vi "GEA2 Serial Dryer Read Write.vi"(0 "Com Chan":u8, 7 "Dryer Status Serial Data In":T1, 11 "error in (no error)":errorcluster) -> (4 "Dryer Status Serial Data":T1, 6 "Read Buffer":string, 8 "Log String":string, 15 "error out":errorcluster)   [LabVIEW 2014]
uses:
  Dryer Wilt/Type Definitions/WILT Dryer Com Port Info.ctl
  Dryer Wilt/Type Definitions/WILT Dryer Status Ctrl.ctl
  Type Definitions/GEA2 Serial Dryer Interface Ctrl.ctl
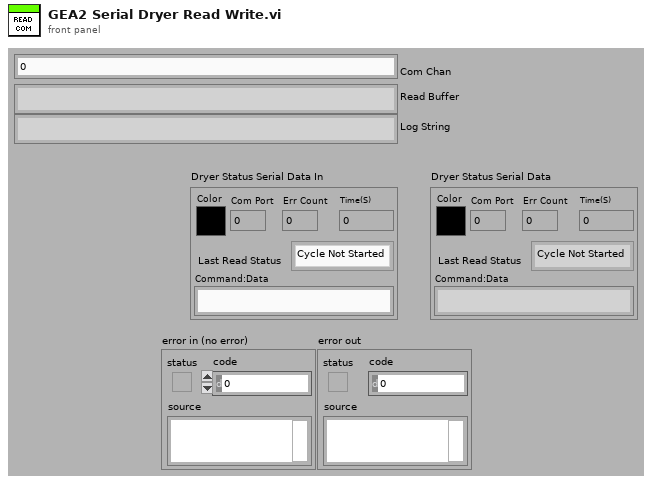
[diagram p1: front panel]
types:
  T1 = typedef "WILT Dryer Com Port Info.ctl" = cluster{"Color":u32, "Last Read Status":T2, "Command:Data":string, "Com Port":u8, "Time(S)":dbl, "Err Count":u32}
  T2 = typedef "WILT Dryer Status Ctrl.ctl" = enum16{"Cycle Not Started", "Cycle Running", "Paused", "Cycle Completed", "Eval Mode Entered", "Err", "Pause (No GEA2)"}
  T3 = typedef "GEA2 Serial Dryer Interface Ctrl.ctl" = enum16{"Init Com Port", "SendCMD", "ReadPort", "Close Port", "Simulate Diag Data", "Send WILT Startup CMDs", "Send Continue CMD", "Read Continuous"}
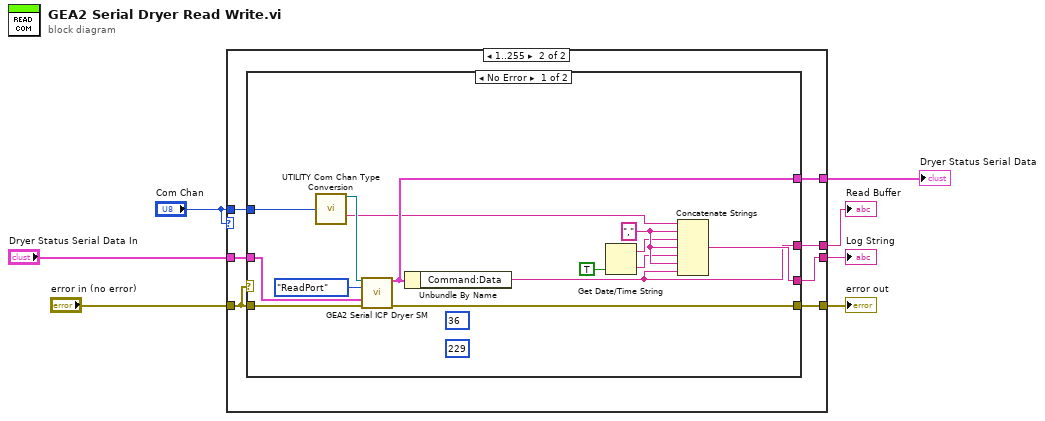
[diagram p0: block diagram]
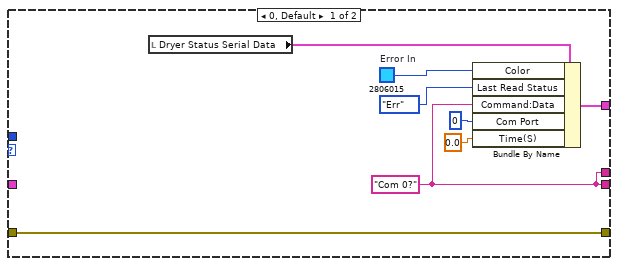
[diagram p2: hidden frame]
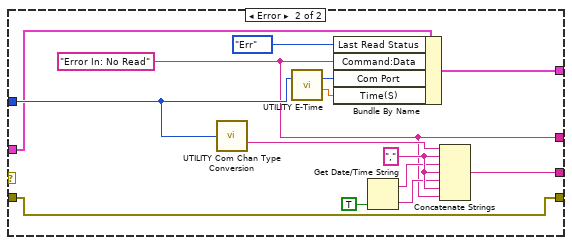
[diagram p3: hidden frame]
diagram:
  n1 = case shown="1..255" "Com Chan" {
    tunnel: "Com Chan" -> [_ w22]
    tunnel: [w15 w21] -> w7
    tunnel: "error in (no error)" -> [w15 w20]
    tunnel: [w11 w19] -> w1
    tunnel: [w11 w18] -> w4
    tunnel: [w8 w17] -> w3
    tunnel: "Dryer Status Serial Data In" -> [_ w16]
    frame 0, Default {
      w12 = u32 2806015  # Error In
      w11 = "Com 0?" ("ASCII Data")
      n2 = local read "Dryer Status Serial Data"() -> (w14:T1)
      n3 = Bundle By Name(cluster=w14, "Color"=w12, "Last Read Status"=WILT_Dryer_Status_Ctrl."Err" ("Status"), "Command:Data"=w11, "Com Port"=u8 0, "Time(S)"=0.0) -> (w8:T1)
    }
    frame 1..255 {
      n4 = case shown="No Error" w20 {
        tunnel: w22 -> [w29 w43]
        tunnel: [w36 w49] -> w21
        tunnel: w20 -> [w35 w49]
        tunnel: [w28 w40] -> w19
        tunnel: [w27 w39] -> w18
        tunnel: [w26 w38] -> w17
        tunnel: w16 -> [w23 w37]
        frame No Error {
          (unwired) u8 36 ("Destination Address")
          (unwired) u8 229 ("Source Address")
          w33 = "," ("string")
          n5 = call "UTILITY Com Chan Type Conversion.vi"("Com Chan"=w29) -> ("VISA resource name"=w34:refnum<visa-resource-name>, "Com Text"=w24:string)  [unwired: 11 in, 2 out]
          n6 = call "GEA2 Serial ICP Dryer SM.vi"("ComPort"=w34, "Mode"=GEA2_Serial_Dryer_Interface_Ctrl."ReadPort", "Dryer Status Serial Data In"=w23, "Error In"=w35) -> ("Dryer Status Serial Data Out"=w26:T1, "Error Out"=w36:errorcluster)  [unwired: 7 in, 3 out]
          n7 = Unbundle By Name(w26) -> ("Command:Data"=w27:string)
          n8 = Get Date/Time String(want seconds? (F)=TRUE) -> (date string=w31:string, time string=w32:string)  [unwired: 2 in]
          n9 = Concatenate Strings(w24, w33, w31, w33, w32, w33, w27) -> (w28:string)
        }
        frame Error {
          w39 = "Error In: No Read" ("ASCII Data")
          w48 = "," ("string")
          n10 = call "UTILITY Com Chan Type Conversion.vi"("Com Chan"=w43) -> ("Com Text"=w44:string)  [unwired: 11 in, 3 out]
          n11 = call "UTILITY E-Time.vi"() -> ("Elapsed Time (sec)"=w41:dbl)  [unwired: 9 in, 2 out]
          n12 = Bundle By Name(cluster=w37, "Last Read Status"=WILT_Dryer_Status_Ctrl."Err" ("Status"), "Command:Data"=w39, "Com Port"=w43, "Time(S)"=w41) -> (w38:T1)
          n13 = Get Date/Time String(want seconds? (F)=TRUE) -> (date string=w46:string, time string=w47:string)  [unwired: 2 in]
          n14 = Concatenate Strings(w44, w48, w46, w48, w47, w48, w39) -> (w40:string)
        }
      }
    }
  }
  "error out" <- w7
  "Log String" <- w1
  "Read Buffer" <- w4
  "Dryer Status Serial Data" <- w3
